vi "Get Initialization Status.vi"(8 "error in (no error)":errorcluster, 11 "RxTx in":refnum<class "RxTx.lvclass">) -> (0 "error out":errorcluster, 3 "RxTx out":refnum<class "RxTx.lvclass">)   [LabVIEW 2018, in "RxTx.lvclass"]
uses:
  RxTx.lvclass
  RxTx.lvclass/RxTx.ctl
  Interface/Interface.lvclass
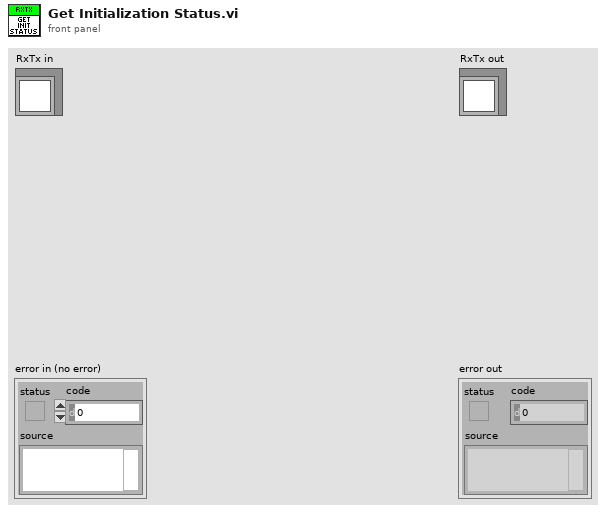
[diagram p1: front panel]
types:
  T1 = cluster{"Initialization":bool, "Serial Number":u16}
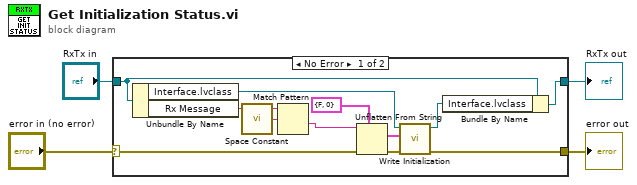
[diagram p0: block diagram]
diagram:
  n1 = case shown="No Error" "error in (no error)" {
    selector: "error in (no error)" -> [w8 w18]
    tunnel: [w7 w18] -> w3
    tunnel: [w5 w17] -> w1
    tunnel: "RxTx in" -> [w6 w17]
    frame No Error {
      n2 = Unbundle By Name(w6) -> ("Interface.lvclass"=w10:refnum<class "Interface.lvclass">, "Rx Message"=w9:string)
      n3 = call <vilib>:"Space Constant.vi"() -> ("String"=w16:string)
      n4 = Match Pattern(string=w9, regular expression=w16) -> (after substring=w15:string)  [unwired: 1 in, 3 out]
      n5 = Unflatten From String(type=T1 {"Initialization"=FALSE, "Serial Number"=0} ("Initialization"), binary string=w15, error in (no error)=w8) -> (value=w11:T1, error out=w13:errorcluster)  [unwired: 2 in, 1 out]
      n6 = call "Write Initialization.vi"("error in (no error)"=w13, "Initialization"=w11, "Interface in"=w10) -> ("error out"=w7:errorcluster, "Interface out"=w14:refnum<class "Interface.lvclass">)  [unwired: 7 in]
      n7 = Bundle By Name(cluster=w6, "Interface.lvclass"=w14) -> (w5:refnum<class "RxTx.lvclass">)
    }
    frame Error {
    }
  }
  "error out" <- w3
  "RxTx out" <- w1
